vi "GEN_SetSettings.vi"(5 "Frequency (1000 Hz)":dbl=1000.0 format="%#.6g", 6 "DC Offset (0.00 V)":dbl, 7 "Amplitude (1.0 Vpp)":dbl=1.0 format="%#.3f", 8 "error in (no error)":errorcluster, 10 "Configuration Cluster":T1={"General"={"Config.ini"=path "", "Default Logging Path"=path ""}, "Hardware"={"Global T VAR"="", "Global B VAR"="", "VISAS"={"GEN COM"="", "SCOPE COM"="", "VNA COM"=""}, "Connected?"={"SCOPE"=FALSE, "GEN"=FALSE, "VNA"=FALSE}}, "Operation"={"Operation Mode"=enum."Idle-Off", "Status"="", "NewLog?"=FALSE, "OvenWarn"=FALSE, "Scope Settings"={"TimeBase"=0.0, "VerticalScale"=4.0, "Channel"=enum."Channel 2"}, "Gen Settings"={"Amplitude"=0.0, "Frequency"=0.0, "Offset"=0.0}}}) -> (0 "error out":errorcluster, 2 "Configuration Cluster Out":T1={"General"={"Config.ini"=path "", "Default Logging Path"=path ""}, "Hardware"={"Global T VAR"="", "Global B VAR"="", "VISAS"={"GEN COM"="", "SCOPE COM"="", "VNA COM"=""}, "Connected?"={"SCOPE"=FALSE, "GEN"=FALSE, "VNA"=FALSE}}, "Operation"={"Operation Mode"=enum."Idle-Off", "Status"="", "NewLog?"=FALSE, "OvenWarn"=FALSE, "Scope Settings"={"TimeBase"=0.0, "VerticalScale"=4.0, "Channel"=enum."Channel 2"}, "Gen Settings"={"Amplitude"=0.0, "Frequency"=0.0, "Offset"=0.0}}})   [LabVIEW 2021]
uses:
  Config_Cluster.ctl
  Mode_Enum.ctl
  <instrlib>/SDG X Series/SDG X Series.lvlib
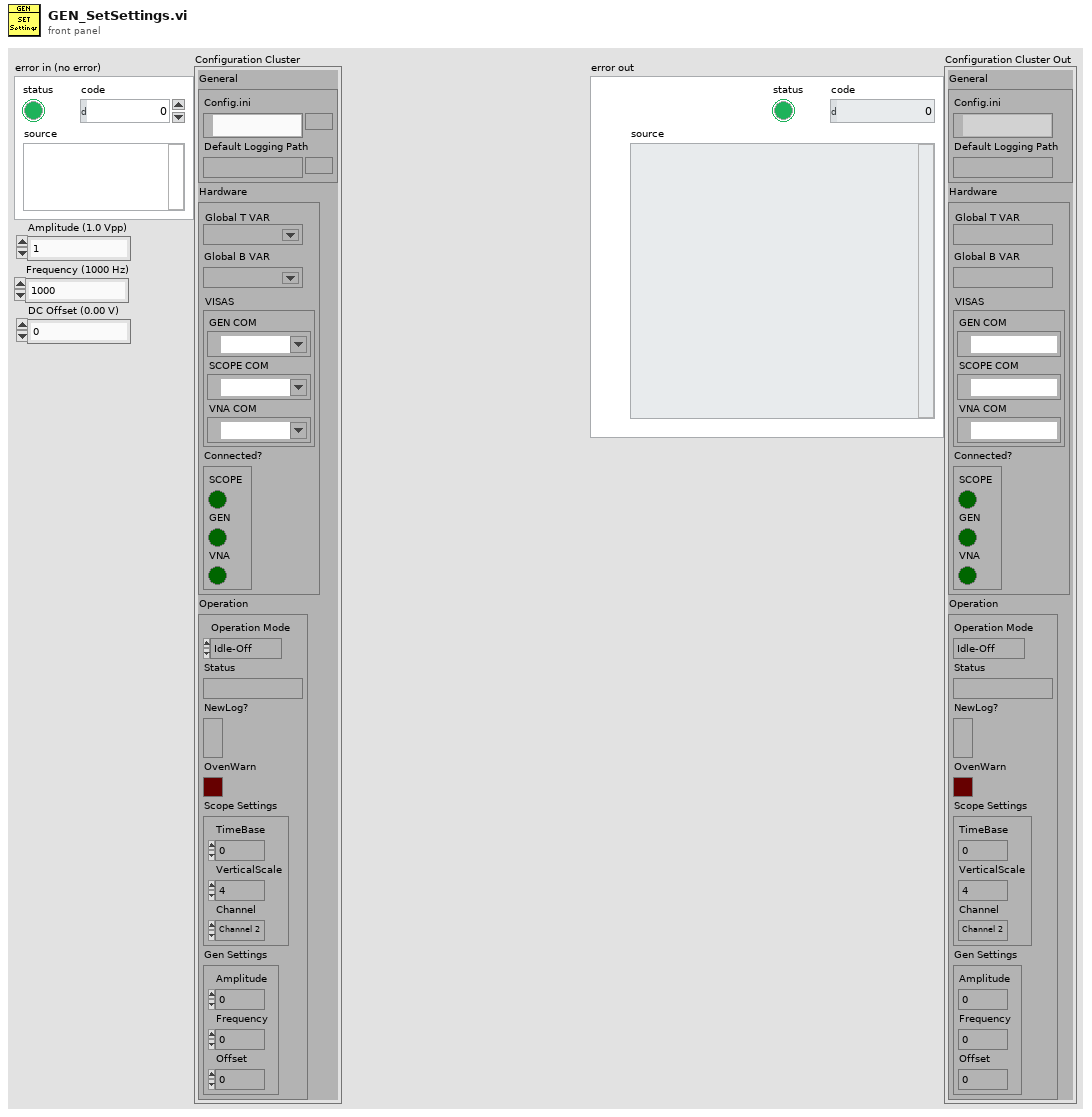
[diagram p1: front panel]
types:
  T1 = typedef "Config_Cluster.ctl" = cluster{"General":cluster{"Config.ini":path, "Default Logging Path":path}, "Hardware":cluster{"Global T VAR":refnum<k21>, "Global B VAR":refnum<k21>, "VISAS":cluster{"GEN COM":refnum<visa-resource-name>, "SCOPE COM":refnum<visa-resource-name>, "VNA COM":refnum<visa-resource-name>}, "Connected?":cluster{"SCOPE":bool, "GEN":bool, "VNA":bool}}, "Operation":cluster{"Operation Mode":T2, "Status":string, "NewLog?":bool, "OvenWarn":bool, "Scope Settings":cluster{"TimeBase":dbl, "VerticalScale":dbl, "Channel":enum16{"Channel 2", "Channel 1"}}, "Gen Settings":cluster{"Amplitude":dbl, "Frequency":dbl, "Offset":dbl}}}
  T2 = typedef "Mode_Enum.ctl" = enum16{"Logging", "Idle-Off", "Idle"}
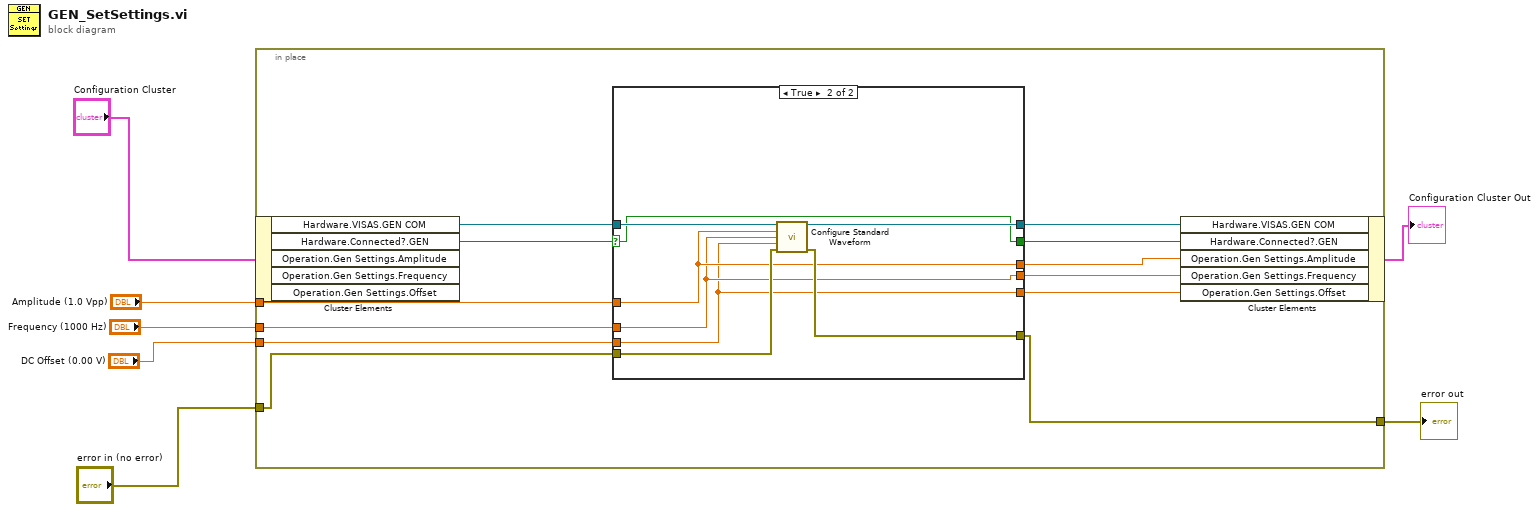
[diagram p0: block diagram]
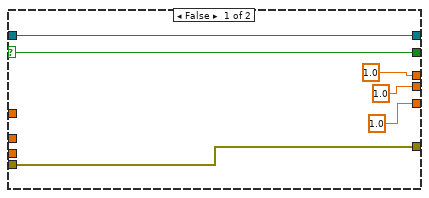
[diagram p2: hidden frame]
diagram:
  n1 = in-place {
    in-place-border: "error in (no error)" -> [w16]
    in-place-border: [w15] -> w4
    in-place-border: "Amplitude (1.0 Vpp)" -> [w11]
    in-place-border: "Frequency (1000 Hz)" -> [w10]
    in-place-border: "DC Offset (0.00 V)" -> [w9]
    n2 = in-place-cluster #1("Configuration Cluster") -> ("Hardware.VISAS.GEN COM"=w18:refnum<visa-resource-name>, "Hardware.Connected?.GEN"=w19:bool)  [unwired: 3 out]
    n3 = case shown="True" w19 {
      selector: w19 -> [w25 w26]
      tunnel: w18 -> [w23 w33]
      tunnel: [w25 w26] -> w17
      tunnel: w16 -> [w24 w31]
      tunnel: [w24 w30] -> w15
      tunnel: [w23 w32] -> w14
      tunnel: [1.0 ("Response Value") w29] -> w13
      tunnel: [1.0 ("Response Value") w28] -> w12
      tunnel: w11 -> [_ w29]
      tunnel: w10 -> [_ w28]
      tunnel: w9 -> [_ w27]
      tunnel: [1.0 ("DC Offset (0.00 V)") w27] -> w8
      frame False {
      }
      frame True {
        n4 = call <instrlib>:"Configure Standard Waveform.vi"("VISA resource name"=w33, "Amplitude (1.0 Vpp)"=w29, "Frequency (1000 Hz)"=w28, "DC Offset (0.00 V)"=w27, "error in (no error)"=w31) -> ("VISA resource name out"=w32:refnum<visa-resource-name>, "error out"=w30:errorcluster)  [unwired: 9 in]
      }
    }
    n5 = in-place-cluster #1("Hardware.VISAS.GEN COM"=w14, "Hardware.Connected?.GEN"=w17, "Operation.Gen Settings.Amplitude"=w13, "Operation.Gen Settings.Frequency"=w12, "Operation.Gen Settings.Offset"=w8) -> (→"Configuration Cluster Out":T1)
  }
  "error out" <- w4
